vi "实时数据查询用2小时间的数据.vi"(11 "字符串":string) -> (3 "连接的字符串":string)   [LabVIEW 2016]
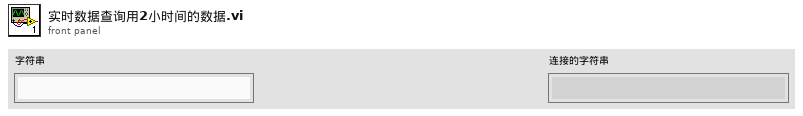
[diagram p1: front panel]
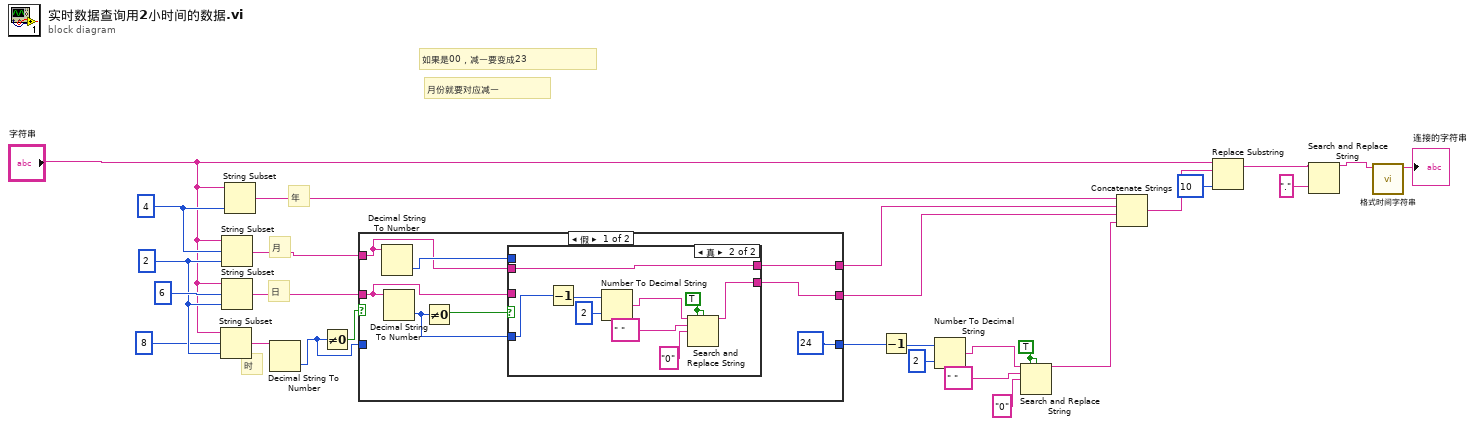
[diagram p0: block diagram]
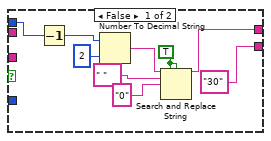
[diagram p2: hidden frame]
diagram:
  w13 = TRUE ("替换全部？(F)")
  w22 = 2 ("长度（剩余）")
  w24 = 4 ("长度（剩余）")
  # "时"
  # "年"
  # "月"
  # "日"
  # "月份就要对应减一"
  # "如果是00，减一要变成23"
  n1 = String Subset(string="字符串", offset (0)=8 ("偏移量(0)"), length (rest)=w22) -> (substring=w19:string)
  n2 = String Subset(string="字符串", offset (0)=w24, length (rest)=w22) -> (substring=w8:string)
  n3 = String Subset(string="字符串", offset (0)=6 ("偏移量(0)"), length (rest)=w22) -> (substring=w9:string)
  n4 = String Subset(string="字符串", length (rest)=w24) -> (substring=w20:string)  [unwired: 1 in]
  n5 = Decimal String To Number(string=w19) -> (number=w17:i32)  [unwired: 2 in, 1 out]
  n6 = Not Equal To 0?(x=w17) -> (x != 0?=w18:bool)
  n7 = case shown="假" w18 {
    tunnel: w17 -> [_ w56]
    tunnel: [24 w56] -> w16
    tunnel: w9 -> [w30 w54]
    tunnel: w8 -> [w29 w55]
    tunnel: [w33 w55] -> w7
    tunnel: [w32 w54] -> w6
    frame False {
      n8 = Decimal String To Number(string=w29) -> (number=w31:i32)  [unwired: 2 in, 1 out]
      n9 = Decimal String To Number(string=w30) -> (number=w28:i32)  [unwired: 2 in, 1 out]
      n10 = Not Equal To 0?(x=w28) -> (x != 0?=w34:bool)
      n11 = case shown="真" w34 {
        tunnel: w31 -> [w43 _]
        tunnel: [w36 w53] -> w33
        tunnel: w30 -> [_ _]
        tunnel: ["30" ("结果字符串") w45] -> w32
        tunnel: w29 -> [_ w53]
        tunnel: w28 -> [_ w46]
        frame False {
          w42 = TRUE ("替换全部？(F)")
          n12 = Decrement(x=w43) -> (x-1=w37:i32)
          n13 = Number To Decimal String(number=w37, width (-)=i16 2 ("宽度(-)")) -> (decimal integer string=w39:string)
          n14 = Search and Replace String(replace all?=w42, case sensitive?=w42, input string=w39, search string=" " ("搜索字符串"), replace string="0" ("替换字符串(\"\")")) -> (result string=w36:string)  [unwired: 3 in, 3 out]
        }
        frame True {
          w49 = TRUE ("替换全部？(F)")
          n15 = Decrement(x=w46) -> (x-1=w48:i32)
          n16 = Number To Decimal String(number=w48, width (-)=i16 2 ("宽度(-)")) -> (decimal integer string=w51:string)
          n17 = Search and Replace String(replace all?=w49, case sensitive?=w49, input string=w51, search string=" " ("搜索字符串"), replace string="0" ("替换字符串(\"\")")) -> (result string=w45:string)  [unwired: 3 in, 3 out]
        }
      }
    }
    frame True {
    }
  }
  n18 = Decrement(x=w16) -> (x-1=w14:i32)
  n19 = Number To Decimal String(number=w14, width (-)=i16 2 ("宽度(-)")) -> (decimal integer string=w11:string)
  n20 = Search and Replace String(replace all?=w13, case sensitive?=w13, input string=w11, search string=" " ("搜索字符串"), replace string="0" ("替换字符串(\"\")")) -> (result string=w5:string)  [unwired: 3 in, 3 out]
  n21 = Concatenate Strings(w20, w7, w6, w5) -> (w4:string)
  n22 = Replace Substring(2:10 ("长度（子字符串长度）"), 4:w4, 5:"字符串") -> (1:w2:string)  [unwired: 1 in, 1 out]
  n23 = Search and Replace String(input string=w2, search string="." ("搜索字符串")) -> (result string=w26:string)  [unwired: 6 in, 3 out]
  n24 = call "格式时间字符串.vi"("字符串"=w26) -> ("连接的字符串"=→"连接的字符串":string)  [unwired: 10 in]
